vi "% to EGU.vi"(1 "coerce output to range? (T)":bool=TRUE, 2 "minimum (EGU)":dbl format="%.2f", 3 "% span":dbl format="%.2f", 4 "maximum (EGU)":dbl format="%.2f") -> (0 "output (EGU)":dbl format="%.2f")   [LabVIEW 2020, in "NI_PID__prctrl compat.lvlib"]
doc: "Converts percent of range input to engineering-units output based upon the min & max range settings. The output is normally limited to the range [max...min]. Values outside of the range [max..min] are allowed when the control coerce output to range? (T) is FALSE."
uses:
  NI_PID__prctrl compat.lvlib
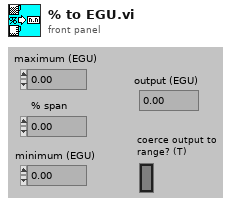
[diagram p1: front panel]
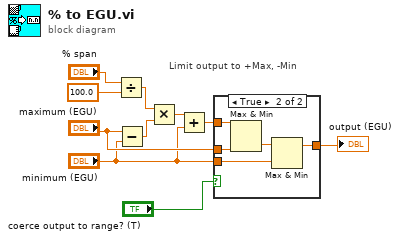
[diagram p0: block diagram]
diagram:
  # "Limit output to +Max, -Min"
  n1 = Divide(x="% span", y=100.0) -> (x/y=w8:dbl)
  n2 = Subtract(x="maximum (EGU)", y="minimum (EGU)") -> (x-y=w7:dbl)
  n3 = Multiply(x=w8, y=w7) -> (x*y=w6:dbl)
  n4 = Add(x=w6, y="minimum (EGU)") -> (x+y=w5:dbl)
  n5 = case shown="True" "coerce output to range? (T)" {
    tunnel: [w11 w16] -> w2
    tunnel: "minimum (EGU)" -> [_ w15]
    tunnel: "maximum (EGU)" -> [_ w13]
    tunnel: w5 -> [w11 w12]
    frame False {
    }
    frame True {
      n6 = Max & Min(x=w12, y=w13) -> (min(x,y)=w14:dbl)  [unwired: 1 out]
      n7 = Max & Min(x=w14, y=w15) -> (max(x,y)=w16:dbl)  [unwired: 1 out]
    }
  }
  "output (EGU)" <- w2
